vi "Write Stamping.vi"(8 "error in (no error)":errorcluster, 10 "Stamping":T1, 11 "Gluing Procedure in":refnum<class "Gluing Procedure.lvclass">) -> (0 "error out":errorcluster, 3 "Gluing Procedure out":refnum<class "Gluing Procedure.lvclass">)   [LabVIEW 2011, in "Gluing Procedure.lvclass"]
uses:
  Gluing Procedure.lvclass
  Type Definitions/Stamping.ctl
  Gluing Procedure.lvclass/Gluing Procedure.ctl
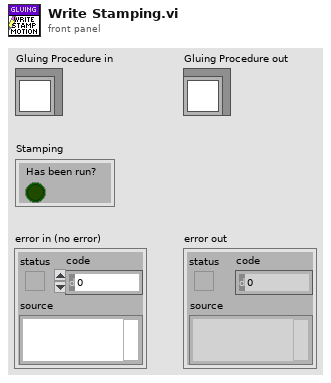
[diagram p1: front panel]
types:
  T1 = typedef "Stamping.ctl" = cluster{"Has been run?":bool}
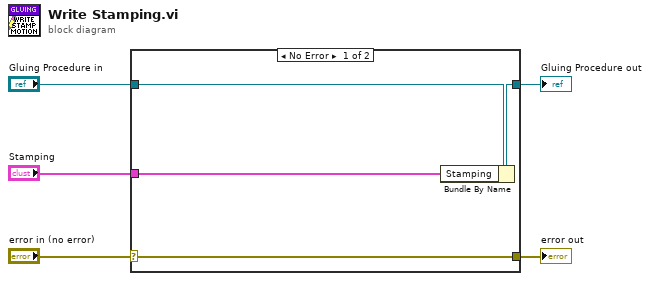
[diagram p0: block diagram]
diagram:
  n1 = case shown="No Error" "error in (no error)" {
    selector: "error in (no error)" -> [w9 w10]
    tunnel: [w9 w10] -> w4
    tunnel: [w7 w11] -> w2
    tunnel: "Gluing Procedure in" -> [w8 w11]
    tunnel: "Stamping" -> [w6 _]
    frame No Error {
      n2 = Bundle By Name(cluster=w8, "Stamping"=w6) -> (w7:refnum<class "Gluing Procedure.lvclass">)
    }
    frame Error {
    }
  }
  "error out" <- w4
  "Gluing Procedure out" <- w2
